vi "VisionAim.vi"(6 "Reset PID":bool, 11 "Angle":dbl=-2.2565641763864366) -> (2 "In Range":bool=TRUE, 3 "Turn Amount":dbl=-0.22037913175901439)   [LabVIEW 2016]
uses:
  Robot Global Data.vi
  Drive Base Class/DriveBase.lvclass
panel:
  in  "Latency":i32=7
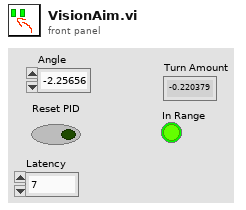
[diagram p1: front panel]
types:
  T1 = cluster{"theta":dbl, "distance":dbl, "x":dbl, "y":dbl}[]
  T2 = cluster{"theta":dbl, "distance":dbl, "x":dbl, "y":dbl}
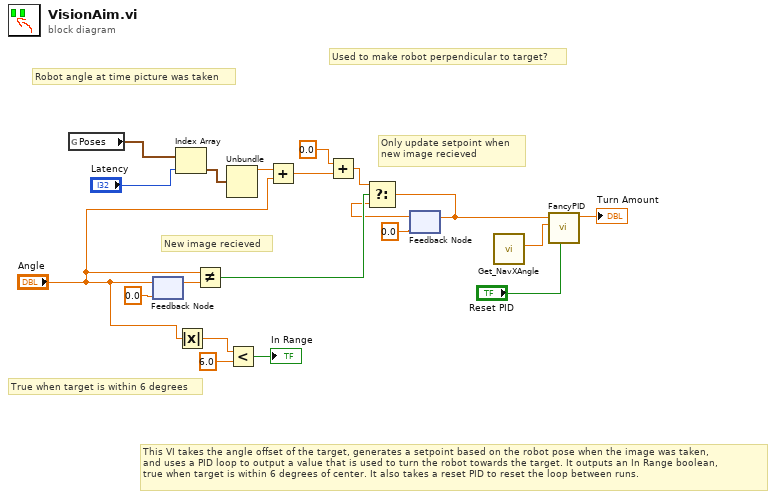
[diagram p0: block diagram]
diagram:
  # "Used to make robot perpendicular to target?"
  # "This VI takes the angle offset of the target, generates a setpoint based on the robot pose when the image was taken,\nand uses a PID loop to output a value that is used to turn the robot towards the target. It outputs an In Range boolean, \ntrue when target is within 6 degrees of center. It also takes a reset PID to reset the loop between runs."
  # "True when target is within 6 degrees"
  # "Only update setpoint when\nnew image recieved"
  # "New image recieved"
  # "Robot angle at time picture was taken"
  n1 = global read "Robot Global Data.vi" "Poses"() -> (w2:T1)
  n2 = feedback #1(0.0 ("Numeric")) -> (w16:dbl)
  n3 = feedback-in #1("Angle") -> ()
  n4 = Index Array(array=w2, index="Latency") -> (element=w18:T2)
  n5 = Absolute Value(x="Angle") -> (abs(x)=w12:dbl)
  n6 = Not Equal?(x="Angle", y=w16) -> (x != y?=w13:bool)
  n7 = Unbundle(w18) -> ("theta"=w7:dbl)  [unwired: 3 out]
  n8 = Less?(x=w12, y=6.0) -> (x < y?=→"In Range":bool)
  n9 = Add(x=w7, y="Angle") -> (x+y=w19:dbl)
  n10 = Add(x=0.0 ("Drive offset"), y=w19) -> (x+y=w9:dbl)
  n11 = feedback #2(0.0) -> (w8:dbl)
  n12 = Select(t=w9, s=w13, f=w8) -> (s? t:f=w5:dbl)
  n13 = feedback-in #2(w5) -> ()
  n14 = call "Get_NavXAngle.vi"() -> ("NavX Angle"=w1:dbl)  [unwired: 10 in, 1 out]
  n15 = call "FancyPID.vi"("Reset PID"="Reset PID", "Process Variable"=w1, "Setpoint"=w5) -> ("Output"=→"Turn Amount":dbl)  [unwired: 8 in]
